vi "Build.vi"(6 "Assembly Type":string, 8 "Position":i32, 9 "XYZTheta":dbl[](array[numeric]), 10 "text file":dbl[][](array[numeric]), 11 "Sensor Dispense in":refnum<class "Sensor Dispense.lvclass">) -> (3 "Sensor Dispense out":refnum<class "Sensor Dispense.lvclass">)   [LabVIEW 2021, in "Sensor Dispense.lvclass"]
uses:
  Projects/Sensor Dispense.lvclass
  C:/Users/HEP/Documents/GitHub/Gantry/UCSB-Gantry-HEP-main/Classes/Routine/Dispense/Dispense.lvclass
  Projects/Sensor Dispense.lvclass/Sensor Dispense.ctl
  <vilib>/Analysis/coordinate.llb/2D Cartesian Coordinate Rotation (Scalar).vi
  <vilib>/Analysis/NI_AALPro.lvlib
panel:
  out "CW/CCW":dbl[](array[numeric])
  out "CW/CCW":dbl[](array[numeric])
  out "endpoints 2":dbl[][](array[numeric])
  out "endpoints":dbl[][](array[numeric])
  out "data":T1(array[cluster])
  out "cell count":dbl[](array[numeric])
  out "centers":dbl[][](array[numeric])
  # "[x1,y1,x2,y2]"
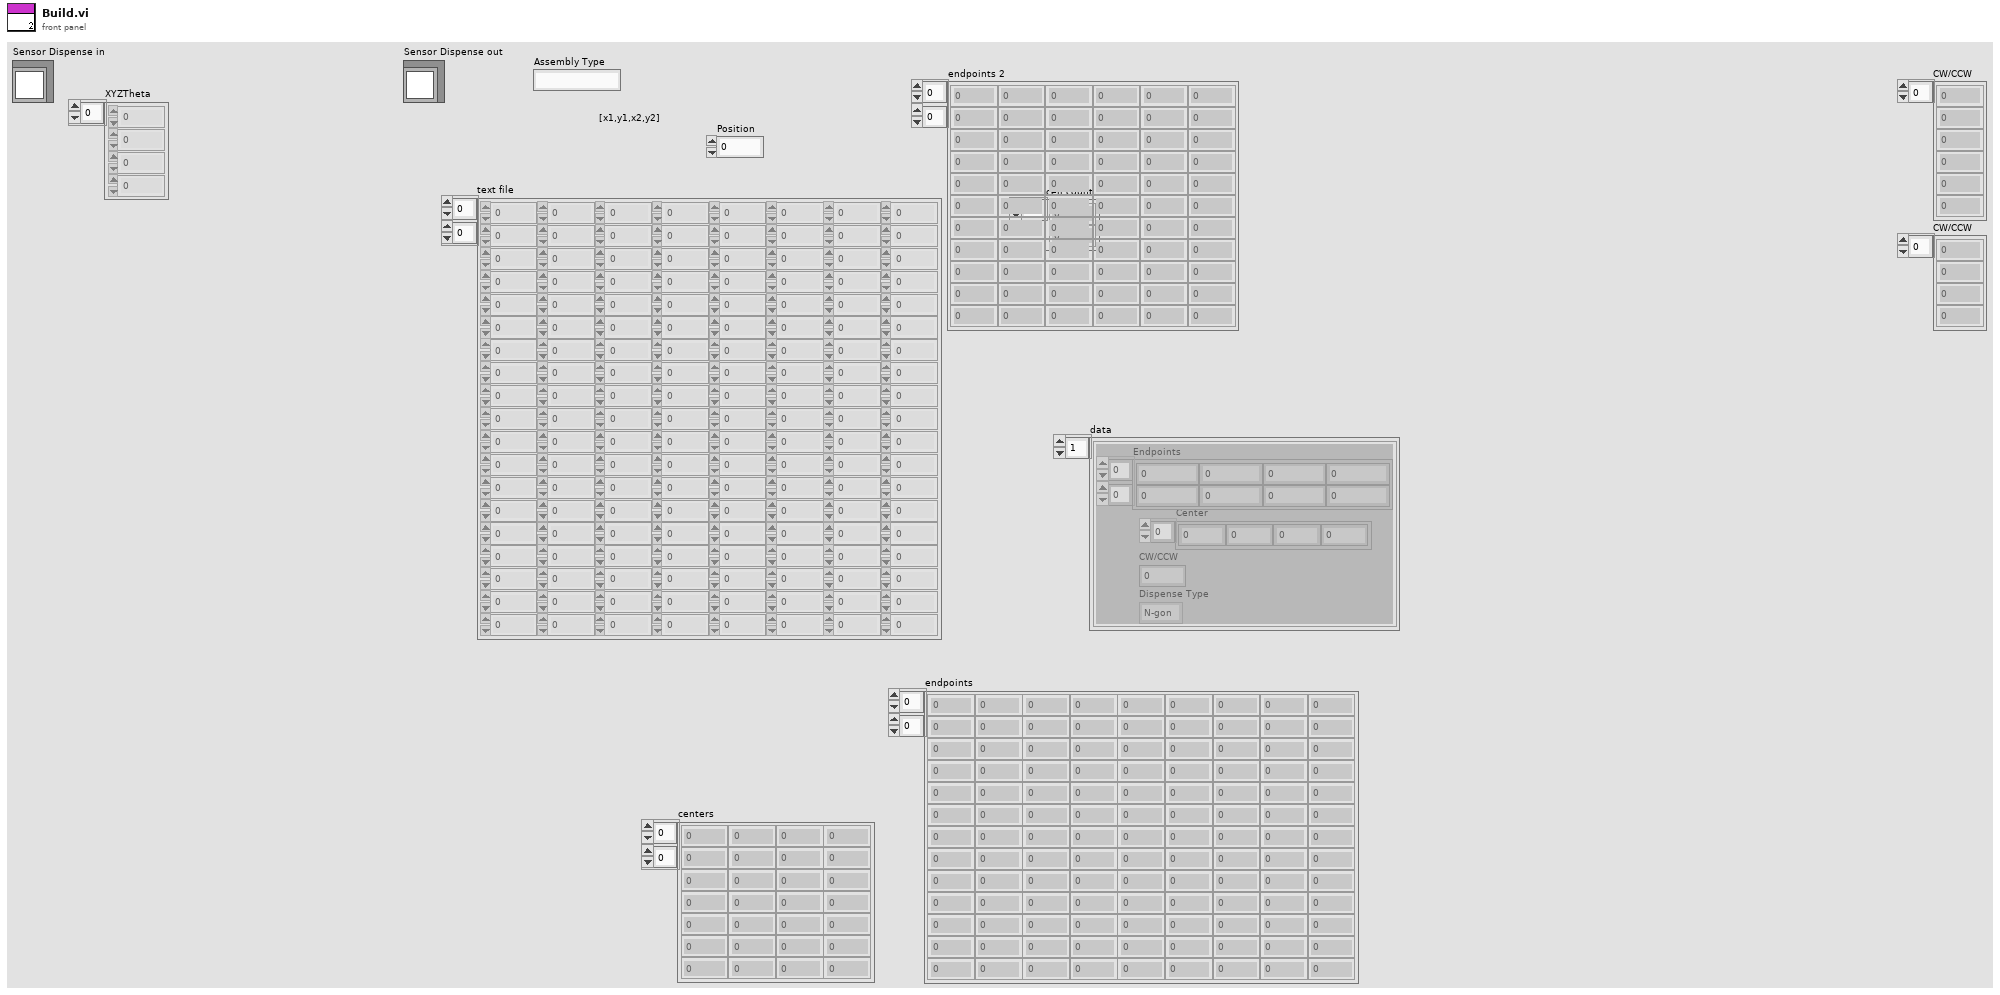
[diagram p1: front panel]
types:
  T1 = cluster{"Endpoints":dbl[][], "Center":dbl[], "CW/CCW":dbl, "Dispense Type":enum16{"N-gon", "Square", "Arc", "Dot", "Line", "Circle"}}[]
  T2 = enum16{"N-gon", "Square", "Arc", "Dot", "Line", "Circle"}
  T3 = cluster{"Endpoints":dbl[][], "Center":dbl[], "CW/CCW":dbl, "Dispense Type":enum16{"N-gon", "Square", "Arc", "Dot", "Line", "Circle"}}
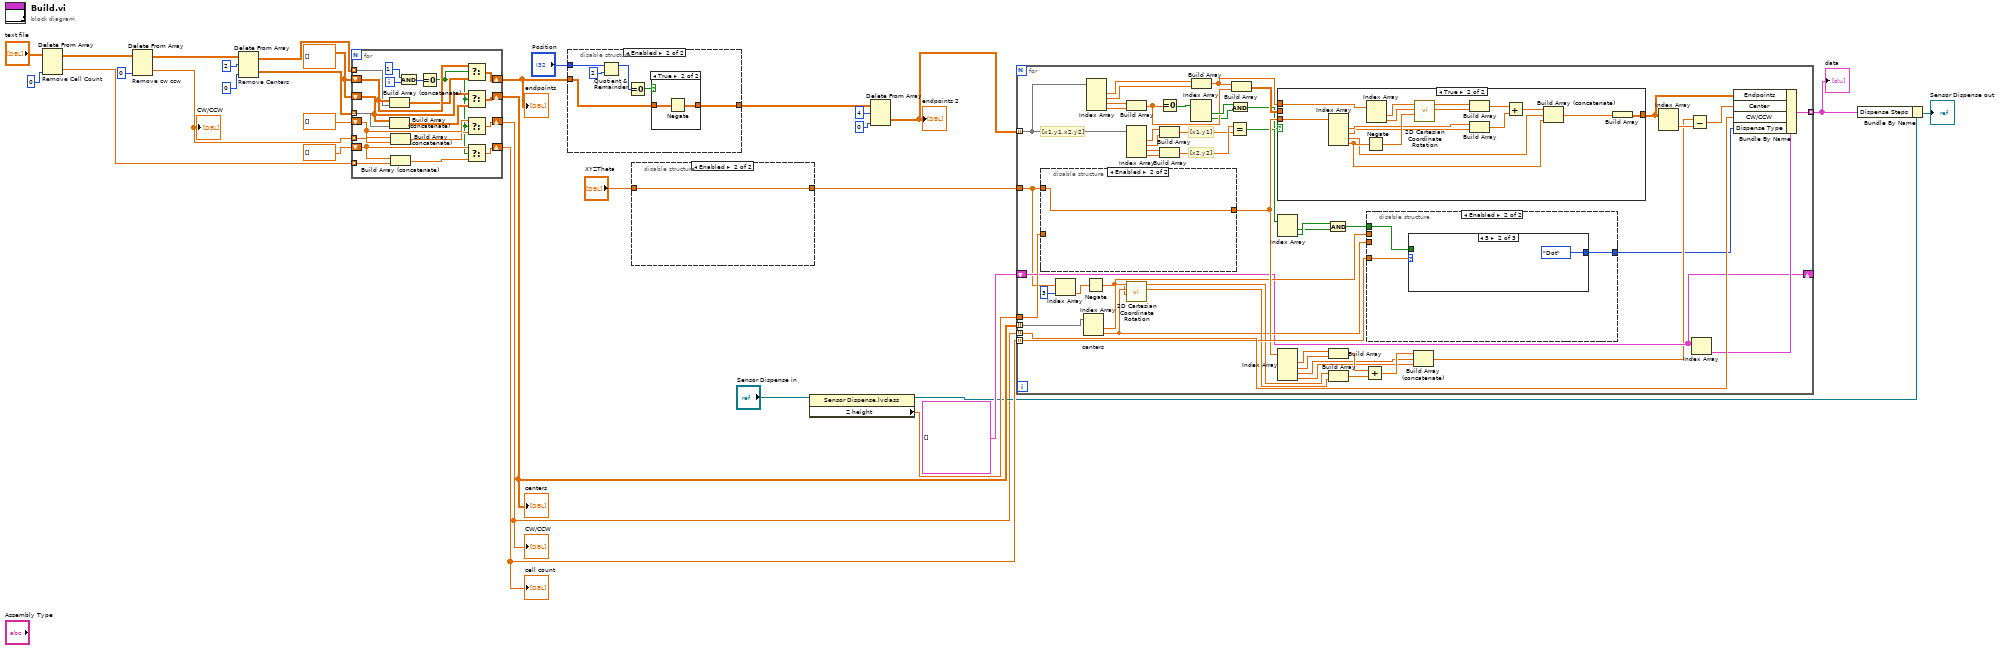
[diagram p0: block diagram]
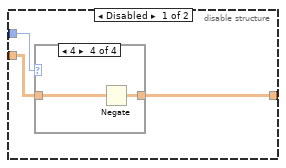
[diagram p2: hidden frame]
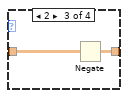
[diagram p5: hidden frame]
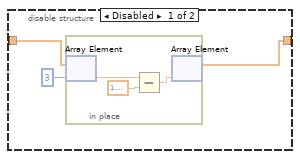
[diagram p7: hidden frame]
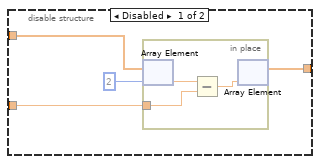
[diagram p8: hidden frame]
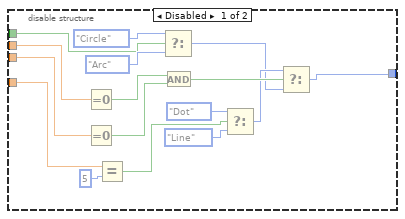
[diagram p9: hidden frame]
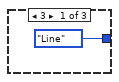
[diagram p10: hidden frame]
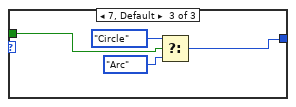
[diagram p11: hidden frame]
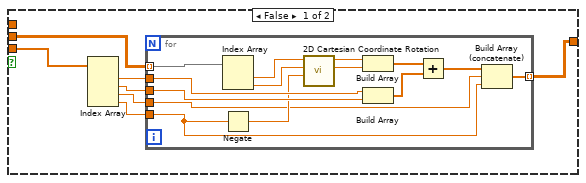
[diagram p12: hidden frame]
diagram:
  w28 = dbl[][] []
  n1 = Delete From Array "Remove Cell Count"(array="text file", index (col)=0) -> (deleted portion=w22:dbl[], array with subset deleted=w24:dbl[][])  [unwired: 2 in]
  n2 = Delete From Array "Remove cw ccw"(array=w24, index (col)=0 ("disabled index (col)")) -> (deleted portion=w5:dbl[], array with subset deleted=w21:dbl[][])  [unwired: 2 in]
  "CW/CCW" <- w5
  n3 = Delete From Array "Remove Centers"(array=w21, length=2, index (col)=0) -> (deleted portion=w17:dbl[][], array with subset deleted=w18:dbl[][])  [unwired: 1 in]
  n4 = for {
    tunnel: w18 -> [w47] mode=indexing
    shift-right: [w45] -> w2
    shift-left: w28 -> [w48]
    tunnel: w17 -> [w44] mode=indexing
    shift-right: [w41] -> w29
    shift-left: w28 -> [w42]
    tunnel: w22 -> [w40] mode=indexing
    shift-right: [w37] -> w26
    shift-left: dbl[] [] -> [w39]
    shift-right: [w32] -> w4
    shift-left: dbl[] [] -> [w35]
    tunnel: w5 -> [w36] mode=indexing
    i -> [w50]
    n5 = Build Array (concatenate)(w48, w47) -> (w46:dbl[][])
    n6 = Build Array (concatenate)(w42, w44) -> (w43:dbl[][])
    n7 = Build Array (concatenate)(w35, w36) -> (w34:dbl[])
    n8 = Build Array (concatenate)(w39, w40) -> (w38:dbl[])
    n9 = And(x=1, y=w50) -> (x .and. y?=w49:i32)
    n10 = Equal To 0?(x=w49) -> (x = 0?=w33:bool)
    n11 = Select(t=w48, s=w33, f=w46) -> (s? t:f=w45:dbl[][])
    n12 = Select(t=w42, s=w33, f=w43) -> (s? t:f=w41:dbl[][])
    n13 = Select(t=w35, s=w33, f=w34) -> (s? t:f=w32:dbl[])
    n14 = Select(t=w39, s=w33, f=w38) -> (s? t:f=w37:dbl[])
  }
  "centers" <- w29
  "cell count" <- w26
  "endpoints" <- w2
  "CW/CCW" <- w4
  n15 = disable-structure shown="Enabled" {
    disable-tunnel: "Position" -> [w54 w66]
    disable-tunnel: [w53 w61] -> w3
    disable-tunnel: w2 -> [w52 w62]
    frame Disabled {
      n16 = case shown="4" w54 {
        tunnel: [w55 w56 w58 w60] -> w53
        tunnel: w52 -> [w55 w56 w57 w59]
        frame 1, Default {
        }
        frame 3 {
        }
        frame 2 {
          n17 = Negate(x=w57) -> (-x=w58:dbl[][])
        }
        frame 4 {
          n18 = Negate(x=w59) -> (-x=w60:dbl[][])
        }
      }
    }
    frame Enabled {
      n19 = Quotient & Remainder(x=w66, y=2) -> (x-y*floor(x/y)=w64:i32)  [unwired: 1 out]
      n20 = Equal To 0?(x=w64) -> (x = 0?=w63:bool)
      n21 = case shown="True" w63 {
        tunnel: w62 -> [w67 w69]
        tunnel: [w67 w68] -> w61
        frame False {
        }
        frame True {
          n22 = Negate(x=w69) -> (-x=w68:dbl[][])
        }
      }
    }
  }
  n23 = disable-structure shown="Enabled" {
    disable-tunnel: "XYZTheta" -> [w72 w76]
    disable-tunnel: [w70 w76] -> w7
    frame Disabled {
      n24 = in-place {
        n25 = in-place-array #1(w72, 3) -> (w75:dbl)
        n26 = Subtract(x=w75, y=1.5707963267948966) -> (x-y=w73:dbl)
        n27 = in-place-array #1(w73) -> (w70:dbl[])  [unwired: 1 out]
      }
    }
    frame Enabled {
    }
  }
  n28 = property class="Sensor Dispense.lvclass"(reference="Sensor Dispense in") -> (reference out=w14:refnum<class "Sensor Dispense.lvclass">, "Z height"=w31:dbl)  [unwired: 1 in, 1 out]
  n29 = Delete From Array(array=w3, length=4, index (col)=0 ("disabled index (col)")) -> (deleted portion=w9:dbl[][])  [unwired: 1 in, 1 out]
  "endpoints 2" <- w9
  n30 = for {
    tunnel: w9 -> [w90] mode=indexing
    tunnel: w7 -> [w99]
    tunnel: w31 -> [w126]
    tunnel: w29 -> [w125] mode=indexing
    tunnel: w4 -> [w124] mode=indexing
    tunnel: w26 -> [w123] mode=indexing
    shift-right: [w108] -> _
    shift-left: T1 [] ("Dispense Steps") -> [w108]
    tunnel: [w122] -> w13 mode=indexing
    # "[x2,y2]"
    # "[x1,y1]"
    # "[x1,y1,x2,y2]"
    n31 = disable-structure shown="Enabled" {
      disable-tunnel: w126 -> [w130 _]
      disable-tunnel: [w129 w134] -> w119
      disable-tunnel: w99 -> [w128 w134]
      frame Disabled {
        n32 = in-place {
          in-place-border: w130 -> [w132]
          n33 = in-place-array #2(w128, 2) -> (w133:dbl)
          n34 = Subtract(x=w133, y=w132) -> (x-y=w131:dbl)
          n35 = in-place-array #2(w131) -> (w129:dbl[])  [unwired: 1 out]
        }
      }
      frame Enabled {
      }
    }
    n36 = Index Array(array=w99, index=3) -> (element=w98:dbl)
    n37 = Index Array "centers"(array=w125) -> (element #1=w111:dbl, element #2=w110:dbl)  [unwired: 2 in]
    n38 = Negate(x=w98) -> (-x=w97:dbl)
    n39 = Index Array(array=w90) -> (element #1=w88:dbl, element #2=w87:dbl, element #3=w86:dbl, element #4=w85:dbl)  [unwired: 4 in]
    n40 = Build Array(w86, w85) -> (w82:dbl[])
    n41 = Index Array(array=w90) -> (element #1=w95:dbl, element #2=w94:dbl, element #3=w107:dbl, element #4=w106:dbl)  [unwired: 4 in]
    n42 = call-poly <vilib>:"2D Cartesian Coordinate Rotation.vi"("theta"=w97, "y"=w110, "x"=w111) -> ("y out"=w120:dbl, "x out"=w121:dbl)  [unwired: 6 in, 1 out]
    n43 = Equal To 0?(x=w82) -> (x = 0?=w81:bool[])
    n44 = Build Array(w95, w94) -> (w104:dbl[])
    n45 = Build Array(w107, w106) -> (w105:dbl[])
    n46 = Index Array(array=w81) -> (element #1=w83:bool, element #2=w79:bool)  [unwired: 2 in]
    n47 = Build Array(w88, w87) -> (w78:dbl[])
    n48 = Equal?(x=w105, y=w104) -> (x = y?=w103:bool[])
    n49 = And(x=w83, y=w79) -> (x .and. y?=w80:bool)
    n50 = Build Array(w78, w82) -> (w84:dbl[][])
    n51 = case shown="True" w80 {
      tunnel: w119 -> [w166 w193]
      tunnel: [w165 w181] -> w77
      tunnel: w84 -> [w164 _]
      tunnel: w78 -> [_ w196]
      frame False {
        n52 = Index Array(array=w166) -> (element #1=w163:dbl, element #2=w162:dbl, element #3=w160:dbl, element #4=w161:dbl)  [unwired: 4 in]
        n53 = for {
          tunnel: w164 -> [w180] mode=indexing
          tunnel: w163 -> [w177]
          tunnel: w162 -> [w176]
          tunnel: [w167] -> w165 mode=indexing
          tunnel: w161 -> [w168]
          tunnel: w160 -> [w169]
          n54 = Index Array(array=w180) -> (element #1=w179:dbl, element #2=w178:dbl)  [unwired: 2 in]
          n55 = Negate(x=w168) -> (-x=w171:dbl)
          n56 = call-poly <vilib>:"2D Cartesian Coordinate Rotation.vi"("theta"=w171, "y"=w178, "x"=w179) -> ("y out"=w174:dbl, "x out"=w175:dbl)  [unwired: 6 in, 1 out]
          n57 = Build Array(w175, w174) -> (w173:dbl[])
          n58 = Build Array(w177, w176) -> (w172:dbl[])
          n59 = Add(x=w173, y=w172) -> (x+y=w170:dbl[])
          n60 = Build Array (concatenate)(w170, w169, w168) -> (w167:dbl[])
        }
      }
      frame True {
        n61 = Index Array(array=w193) -> (element #1=w189:dbl, element #2=w188:dbl, element #3=w184:dbl, element #4=w185:dbl)  [unwired: 4 in]
        n62 = Negate(x=w185) -> (-x=w192:dbl)
        n63 = Index Array(array=w196) -> (element #1=w195:dbl, element #2=w194:dbl)  [unwired: 2 in]
        n64 = call-poly <vilib>:"2D Cartesian Coordinate Rotation.vi"("theta"=w192, "y"=w194, "x"=w195) -> ("y out"=w190:dbl, "x out"=w191:dbl)  [unwired: 6 in, 1 out]
        n65 = Build Array(w191, w190) -> (w186:dbl[])
        n66 = Build Array(w189, w188) -> (w187:dbl[])
        n67 = Add(x=w186, y=w187) -> (x+y=w183:dbl[])
        n68 = Build Array (concatenate)(w183, w184, w185) -> (w182:dbl[])
        n69 = Build Array(w182) -> (w181:dbl[][])
      }
    }
    n70 = Index Array(array=w103) -> (element #1=w101:bool, element #2=w102:bool)  [unwired: 2 in]
    n71 = Index Array(array=w119) -> (element #1=w118:dbl, element #2=w115:dbl, element #3=w113:dbl, element #4=w112:dbl)  [unwired: 4 in]
    n72 = And(x=w102, y=w101) -> (x .and. y?=w100:bool)
    n73 = Build Array(w118, w115) -> (w117:dbl[])
    n74 = Build Array(w121, w120) -> (w116:dbl[])
    n75 = Add(x=w117, y=w116) -> (x+y=w114:dbl[])
    n76 = disable-structure shown="Enabled" {
      disable-tunnel: w123 -> [w150 w153]
      disable-tunnel: w111 -> [w147 _]
      disable-tunnel: w110 -> [w146 _]
      disable-tunnel: w100 -> [w139 w152]
      disable-tunnel: [w135 w151] -> w89
      frame Disabled {
        n77 = Equal To 0?(x=w147) -> (x = 0?=w148:bool)
        n78 = Equal To 0?(x=w146) -> (x = 0?=w149:bool)
        n79 = Equal?(x=w150, y=5) -> (x = y?=w142:bool)
        n80 = Select(t=T2."Circle" ("Dispense Type"), s=w139, f=T2."Arc" ("Dispense Type")) -> (s? t:f=w136:T2)
        n81 = And(x=w148, y=w149) -> (x .and. y?=w138:bool)
        n82 = Select(t=T2."Dot" ("Dispense Type"), s=w142, f=T2."Line" ("Dispense Type")) -> (s? t:f=w137:T2)
        n83 = Select(t=w137, s=w138, f=w136) -> (s? t:f=w135:T2)
      }
      frame Enabled {
        n84 = case shown="5" w153 {
          tunnel: w152 -> [_ _ w157]
          tunnel: [T2."Line" ("Dispense Type") T2."Dot" ("Dispense Type") w156] -> w151
          frame 3 {
          }
          frame 5 {
          }
          frame 7, Default {
            n85 = Select(t=T2."Circle" ("Dispense Type"), s=w157, f=T2."Arc" ("Dispense Type")) -> (s? t:f=w156:T2)
          }
        }
      }
    }
    n86 = Build Array (concatenate)(w114, w113, w112) -> (w92:dbl[])
    n87 = Index Array(array=w77) -> (element=w93:dbl[])  [unwired: 2 in]
    n88 = Subtract(x=w92, y=w93) -> (x-y=w91:dbl[])
    n89 = Index Array(array=w108) -> (element=w109:T3)  [unwired: 1 in]
    n90 = Bundle By Name(cluster=w109, "Endpoints"=w77, "Center"=w91, "CW/CCW"=w124, "Dispense Type"=w89) -> (w122:T3)
  }
  "data" <- w13
  n91 = Bundle By Name(cluster=w14, "Dispense Steps"=w13) -> (→"Sensor Dispense out":refnum<class "Sensor Dispense.lvclass">)
